vi "raster_scan_ground_shutter_new1.vi"() -> ()   [LabVIEW 2014] (continued)
{"X"=1085.0, "Y"=1.0008017239957097}, {"X"=1086.0, "Y"=1.0006641645030927}, {"X"=1087.0, "Y"=1.0004027285217332}, {"X"=1088.0, "Y"=1.0005489411934159}, {"X"=1089.0, "Y"=1.0007225000918056}, {"X"=1090.0, "Y"=1.0009034474609535}, {"X"=1091.0, "Y"=1.000700412495902}, {"X"=1092.0, "Y"=1.000559530919639}, {"X"=1093.0, "Y"=1.000504483593376}, {"X"=1094.0, "Y"=1.0006442407338632}, {"X"=1095.0, "Y"=1.0007664841012642}, {"X"=1096.0, "Y"=1.000595386528809}, {"X"=1097.0, "Y"=1.0006037218552855}, {"X"=1098.0, "Y"=1.0006076992023385}, {"X"=1099.0, "Y"=1.0008559458938961}, {"X"=1100.0, "Y"=1.0003974508855653}, {"X"=1101.0, "Y"=1.000520661832493}, {"X"=1102.0, "Y"=1.0007578111149742}, {"X"=1103.0, "Y"=1.0008950719357999}, {"X"=1104.0, "Y"=1.0005845587993554}, {"X"=1105.0, "Y"=1.0004975573787183}, {"X"=1106.0, "Y"=1.0005630280187985}, {"X"=1107.0, "Y"=1.0004865609128089}, {"X"=1108.0, "Y"=1.0005512637747156}, {"X"=1109.0, "Y"=1.0002904477140733}, {"X"=1110.0, "Y"=1.0007674753310123}, {"X"=1111.0, "Y"=1.00048425912666}, {"X"=1112.0, "Y"=1.000537310412031}, {"X"=1113.0, "Y"=1.0003184257671687}, {"X"=1114.0, "Y"=1.000551378960108}, {"X"=1115.0, "Y"=1.0004538385686341}, {"X"=1116.0, "Y"=1.0004718054037691}, {"X"=1117.0, "Y"=1.0005247856359447}, {"X"=1118.0, "Y"=1.000659286030276}, {"X"=1119.0, "Y"=1.0005952741982334}, {"X"=1120.0, "Y"=1.0003527948470332}, {"X"=1121.0, "Y"=1.0003785102284437}, {"X"=1122.0, "Y"=1.0003192400893162}, {"X"=1123.0, "Y"=1.0003699743364536}, {"X"=1124.0, "Y"=1.0004382463116217}, {"X"=1125.0, "Y"=1.0006464169345477}, {"X"=1126.0, "Y"=1.000249392202887}, {"X"=1127.0, "Y"=1.0003913257192574}, {"X"=1128.0, "Y"=1.0002131029939758}, {"X"=1129.0, "Y"=1.000510325890708}, {"X"=1130.0, "Y"=1.0003934905817833}, {"X"=1131.0, "Y"=1.0004037059793067}, {"X"=1132.0, "Y"=1.0006618492578454}, {"X"=1133.0, "Y"=1.0003001585452074}, {"X"=1134.0, "Y"=1.000318694948343}, {"X"=1135.0, "Y"=1.000487815893616}, {"X"=1136.0, "Y"=1.0003780216915208}, {"X"=1137.0, "Y"=1.000413317598835}, {"X"=1138.0, "Y"=1.0002135307505462}, {"X"=1139.0, "Y"=1.0003336207033005}, {"X"=1140.0, "Y"=1.000519988073343}, {"X"=1141.0, "Y"=1.000548679843787}, {"X"=1142.0, "Y"=1.000496056734601}, {"X"=1143.0, "Y"=1.0004444345976555}, {"X"=1144.0, "Y"=1.0001817232823744}, {"X"=1145.0, "Y"=1.000174005105797}, {"X"=1146.0, "Y"=1.000292447162328}, {"X"=1147.0, "Y"=1.0003638645546393}, {"X"=1148.0, "Y"=1.0002355752060164}, {"X"=1149.0, "Y"=1.00033455515827}, {"X"=1150.0, "Y"=1.0003245306564827}, {"X"=1151.0, "Y"=1.0002618152857234}, {"X"=1152.0, "Y"=1.0002737777366781}, {"X"=1153.0, "Y"=1.0002170643978059}, {"X"=1154.0, "Y"=1.000413604154719}, {"X"=1155.0, "Y"=1.0003099390465664}, {"X"=1156.0, "Y"=1.0005132182782912}, {"X"=1157.0, "Y"=1.000114107216987}, {"X"=1158.0, "Y"=1.0004770062354829}, {"X"=1159.0, "Y"=1.0004171034572575}, {"X"=1160.0, "Y"=1.0004569184938314}, {"X"=1161.0, "Y"=1.0004500384099237}, {"X"=1162.0, "Y"=1.0003170786145168}, {"X"=1163.0, "Y"=1.0002788252400026}, {"X"=1164.0, "Y"=1.0001948307072348}, {"X"=1165.0, "Y"=1.000410823030397}, {"X"=1166.0, "Y"=1.0004580665102198}, {"X"=1167.0, "Y"=1.0006692310587075}, {"X"=1168.0, "Y"=1.0003228737956749}, {"X"=1169.0, "Y"=1.0004916680510918}, {"X"=1170.0, "Y"=1.0003407364670853}, {"X"=1171.0, "Y"=1.0004045567333217}, {"X"=1172.0, "Y"=1.0003803654908978}, {"X"=1173.0, "Y"=1.0005615371076164}, {"X"=1174.0, "Y"=1.0004756109300434}, {"X"=1175.0, "Y"=1.0002314936984527}, {"X"=1176.0, "Y"=1.0004712973824592}, {"X"=1177.0, "Y"=1.0004057411969836}, {"X"=1178.0, "Y"=1.000628559692479}, {"X"=1179.0, "Y"=1.0003217635313526}, {"X"=1180.0, "Y"=1.0005789076417058}, {"X"=1181.0, "Y"=1.0004029462741326}, {"X"=1182.0, "Y"=1.0004755736162572}, {"X"=1183.0, "Y"=1.000328213200497}, {"X"=1184.0, "Y"=1.0003231498600846}, {"X"=1185.0, "Y"=1.000319103874417}, {"X"=1186.0, "Y"=1.0003228774765789}, {"X"=1187.0, "Y"=1.0003140546407656}, {"X"=1188.0, "Y"=1.0002848343336417}, {"X"=1189.0, "Y"=1.000508203882091}, {"X"=1190.0, "Y"=1.0002593068654488}, {"X"=1191.0, "Y"=1.000528935806764}, {"X"=1192.0, "Y"=1.0002378049460148}, {"X"=1193.0, "Y"=1.0005706812105148}, {"X"=1194.0, "Y"=1.0005374034632506}, {"X"=1195.0, "Y"=1.0001988163757602}, {"X"=1196.0, "Y"=1.0006119463054979}, {"X"=1197.0, "Y"=1.0004849225241381}, {"X"=1198.0, "Y"=1.0001640223128738}, {"X"=1199.0, "Y"=1.000498524564885}, {"X"=1200.0, "Y"=1.0004647778536588}, {"X"=1201.0, "Y"=1.000694727887658}, {"X"=1202.0, "Y"=1.0005207959941573}, {"X"=1203.0, "Y"=1.0004819931045297}, {"X"=1204.0, "Y"=1.000408028714742}, {"X"=1205.0, "Y"=1.000452772334067}, {"X"=1206.0, "Y"=1.0004315291178194}, {"X"=1207.0, "Y"=1.000614562289016}, {"X"=1208.0, "Y"=1.0004267608269495}, {"X"=1209.0, "Y"=1.0005413247966406}, {"X"=1210.0, "Y"=1.0003336212758853}, {"X"=1211.0, "Y"=1.0005233093467742}, {"X"=1212.0, "Y"=1.0001841951286268}, {"X"=1213.0, "Y"=1.000496276064622}, {"X"=1214.0, "Y"=1.0004435113554953}, {"X"=1215.0, "Y"=1.000312762889553}, {"X"=1216.0, "Y"=1.0003880506852765}, {"X"=1217.0, "Y"=1.0004430152993407}, {"X"=1218.0, "Y"=1.0005048604950806}, {"X"=1219.0, "Y"=1.0005918812246315}, {"X"=1220.0, "Y"=1.0005451398371954}, {"X"=1221.0, "Y"=1.0003538628812572}, {"X"=1222.0, "Y"=1.0002957581328165}, {"X"=1223.0, "Y"=1.0003455069942162}, {"X"=1224.0, "Y"=1.000559760984321}, {"X"=1225.0, "Y"=1.0006259813372131}, {"X"=1226.0, "Y"=1.0005780148556396}, {"X"=1227.0, "Y"=1.000428860631512}, {"X"=1228.0, "Y"=1.0003284274537925}, {"X"=1229.0, "Y"=1.0003759087401576}, {"X"=1230.0, "Y"=1.0004160325486642}, {"X"=1231.0, "Y"=1.000516966469858}, {"X"=1232.0, "Y"=1.0003531105538244}, {"X"=1233.0, "Y"=1.0003040660663642}, {"X"=1234.0, "Y"=1.0002145369130029}, {"X"=1235.0, "Y"=1.0006000845056313}, {"X"=1236.0, "Y"=1.0001780143915535}, {"X"=1237.0, "Y"=1.000413099776387}, {"X"=1238.0, "Y"=1.000340814364807}, {"X"=1239.0, "Y"=1.0003847961728747}, {"X"=1240.0, "Y"=1.0003377689644548}, {"X"=1241.0, "Y"=1.000235110479406}, {"X"=1242.0, "Y"=1.0003788090882357}, {"X"=1243.0, "Y"=1.0002683715599725}, {"X"=1244.0, "Y"=1.0005668734989672}, {"X"=1245.0, "Y"=1.0003983214098358}, {"X"=1246.0, "Y"=1.0004392908564488}, {"X"=1247.0, "Y"=1.0003490703578124}, {"X"=1248.0, "Y"=1.000515061423131}, {"X"=1249.0, "Y"=1.000536082836616}, {"X"=1250.0, "Y"=1.0006033938395056}, {"X"=1251.0, "Y"=1.000302436999363}, {"X"=1252.0, "Y"=1.0003435968686736}, {"X"=1253.0, "Y"=1.0003651518565015}, {"X"=1254.0, "Y"=1.0003753816897634}, {"X"=1255.0, "Y"=1.0004164707875218}, {"X"=1256.0, "Y"=1.0003124339083862}, {"X"=1257.0, "Y"=1.0006060617434724}, {"X"=1258.0, "Y"=1.0002433038607497}, {"X"=1259.0, "Y"=1.0005616162726159}, {"X"=1260.0, "Y"=1.0001358996051335}, {"X"=1261.0, "Y"=1.0004996326881244}, {"X"=1262.0, "Y"=1.000400823722666}, {"X"=1263.0, "Y"=1.0004651302016123}, {"X"=1264.0, "Y"=1.0004929661841928}, {"X"=1265.0, "Y"=1.000289786751315}, {"X"=1266.0, "Y"=1.0007068294577364}, {"X"=1267.0, "Y"=1.000512591719354}, {"X"=1268.0, "Y"=1.0005384306699427}, {"X"=1269.0, "Y"=1.000517410690437}, {"X"=1270.0, "Y"=1.0004457834676075}, {"X"=1271.0, "Y"=1.0003882566144624}, {"X"=1272.0, "Y"=1.000350183325496}, {"X"=1273.0, "Y"=1.0006835941128598}, {"X"=1274.0, "Y"=1.000354784112539}, {"X"=1275.0, "Y"=1.0005457804752032}, {"X"=1276.0, "Y"=1.0004234559458807}, {"X"=1277.0, "Y"=1.000496135909765}, {"X"=1278.0, "Y"=1.0002670384407588}, {"X"=1279.0, "Y"=1.0006040819275774}, {"X"=1280.0, "Y"=1.0002955765486259}, {"X"=1281.0, "Y"=1.000449882926412}, {"X"=1282.0, "Y"=1.000341046704705}, {"X"=1283.0, "Y"=1.0002621866108508}, {"X"=1284.0, "Y"=1.0002533451242017}, {"X"=1285.0, "Y"=1.0005020999666248}, {"X"=1286.0, "Y"=1.0004683221869657}, {"X"=1287.0, "Y"=1.0001189169044085}, {"X"=1288.0, "Y"=1.000394207742366}, {"X"=1289.0, "Y"=1.0004025113742172}, {"X"=1290.0, "Y"=1.0003591461387191}, {"X"=1291.0, "Y"=1.0002694424348582}, {"X"=1292.0, "Y"=1.000211944479205}, {"X"=1293.0, "Y"=1.0004554645660035}, {"X"=1294.0, "Y"=1.0004598057481355}, {"X"=1295.0, "Y"=1.0003228478676573}, {"X"=1296.0, "Y"=1.000281777127627}, {"X"=1297.0, "Y"=1.0003787502855446}, {"X"=1298.0, "Y"=1.0002643271177996}, {"X"=1299.0, "Y"=1.0003769449091497}, {"X"=1300.0, "Y"=1.0002871629718717}, {"X"=1301.0, "Y"=1.0002870790211043}, {"X"=1302.0, "Y"=1.0004704503723805}, {"X"=1303.0, "Y"=1.000476260657746}, {"X"=1304.0, "Y"=1.0004436163087576}, {"X"=1305.0, "Y"=1.0003863290955655}, {"X"=1306.0, "Y"=1.0005161647862937}, {"X"=1307.0, "Y"=1.0002249935131708}, {"X"=1308.0, "Y"=1.0005432839193034}, {"X"=1309.0, "Y"=1.0002816770022227}, {"X"=1310.0, "Y"=1.0004166737347884}, {"X"=1311.0, "Y"=1.000377784099795}, {"X"=1312.0, "Y"=1.000352088235326}, {"X"=1313.0, "Y"=1.0002378301300934}, {"X"=1314.0, "Y"=1.0004637548937716}, {"X"=1315.0, "Y"=1.0005468342453412}, {"X"=1316.0, "Y"=1.0002633492264565}, {"X"=1317.0, "Y"=1.000564439873648}, {"X"=1318.0, "Y"=1.0001624654733714}, {"X"=1319.0, "Y"=1.000511231090866}, {"X"=1320.0, "Y"=1.0003544601208683}, {"X"=1321.0, "Y"=1.0004053585602486}, {"X"=1322.0, "Y"=1.0004871315290047}, {"X"=1323.0, "Y"=1.0004300315929238}, {"X"=1324.0, "Y"=1.0003519445352231}, {"X"=1325.0, "Y"=1.0001932579752508}, {"X"=1326.0, "Y"=1.0004275604256458}, {"X"=1327.0, "Y"=1.0004909106276227}, {"X"=1328.0, "Y"=1.0003410593503033}, {"X"=1329.0, "Y"=1.0004439501902358}, {"X"=1330.0, "Y"=1.0005001161868323}, {"X"=1331.0, "Y"=1.0003332716770454}, {"X"=1332.0, "Y"=1.0005933376920328}, {"X"=1333.0, "Y"=1.0002798326870992}, {"X"=1334.0, "Y"=1.0004522633871564}, {"X"=1335.0, "Y"=1.0003822332936998}, {"X"=1336.0, "Y"=1.000511062012222}, {"X"=1337.0, "Y"=1.000358823903489}, {"X"=1338.0, "Y"=1.0006280323541772}, {"X"=1339.0, "Y"=1.00037812862855}]
  in  "# Images":u16=200 min=2 max=10000 step=2
  out "error out":errorcluster
  out "Camera Handle":u32=16842752
  out "Temperature":dbl=-75.5
  in  "error in":errorcluster
  # "Delay Stage Control"
  # "Calibration parameters"
  # "File Destination"
  # "Raster Scan Parameters"
  # "Microscope Stage Control"
  # "Fitting Parameters"
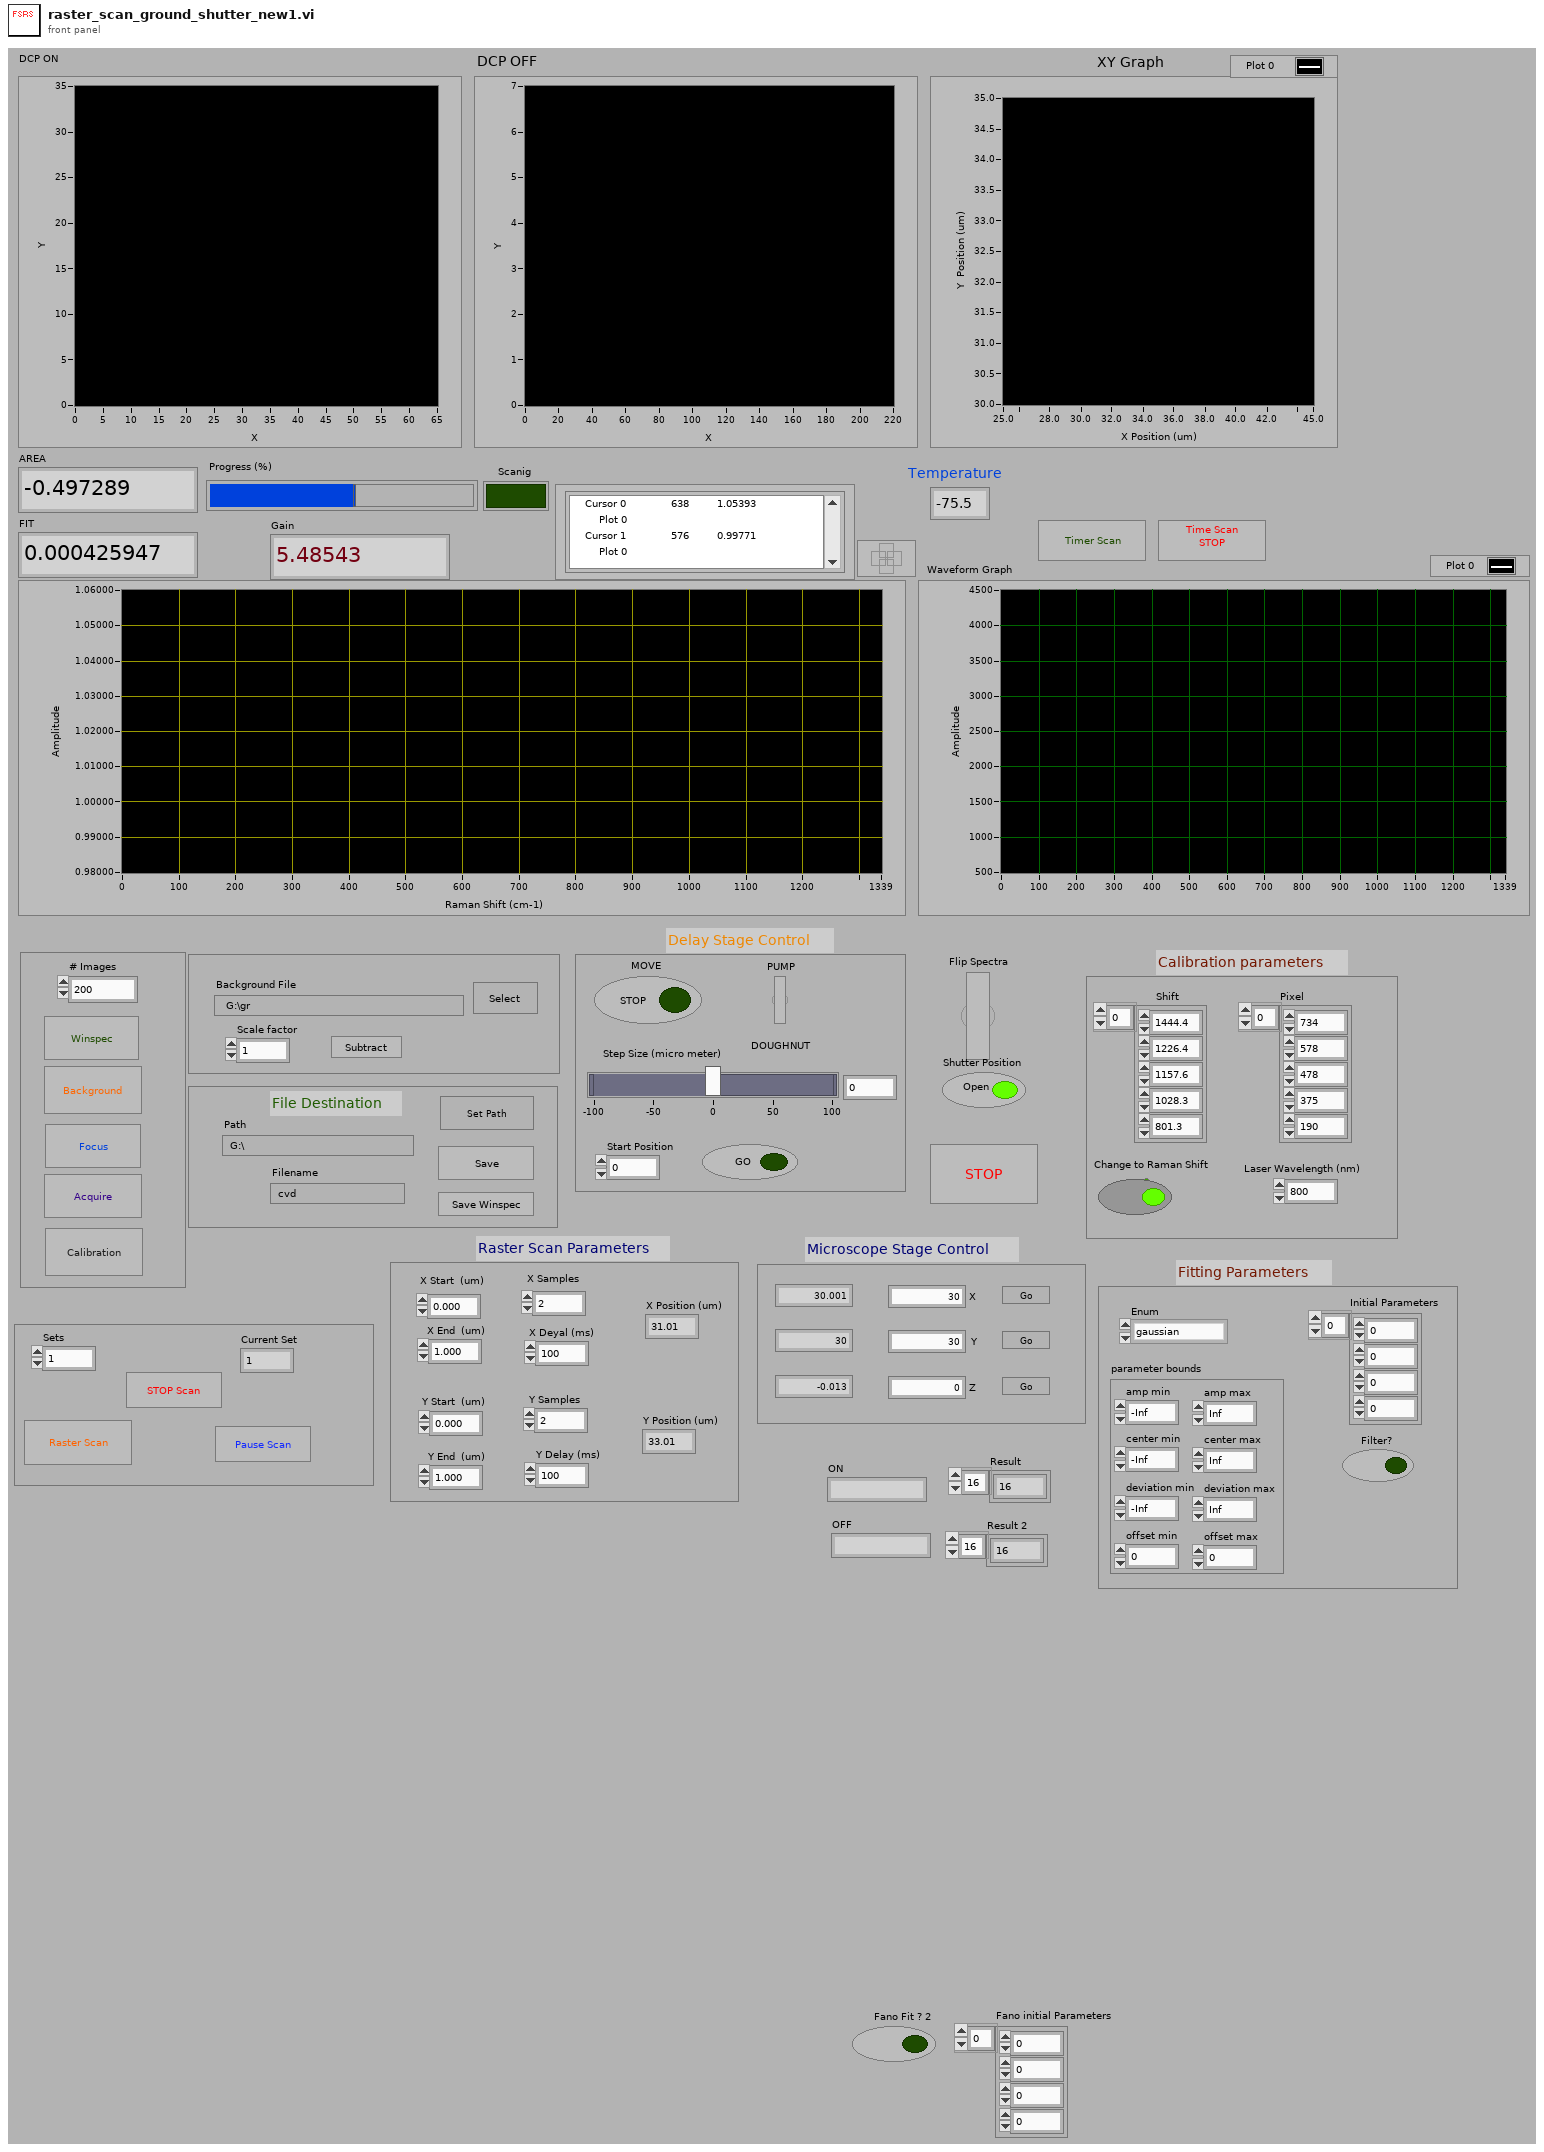
[diagram p1: front panel]
types:
  T1 = cluster{"amp min":dbl, "amp max":dbl, "center min":dbl, "center max":dbl, "deviation min":dbl, "deviation max":dbl, "offset min":dbl, "offset max":dbl}
  T2 = typedef "Control 2.ctl" = dbl[]
  T3 = enum8{"Enabled", "Disabled", "Disabled and Grayed Out"}
  T4 = cluster{"X start":u32, "X end":u32, "X Binning/Grouping":u32, "Y start":u32, "Y end":u32, "Y Binning/Grouping":u32}
  T5 = cluster{dbl[][], dbl[][], dbl[][], dbl[][], bool}
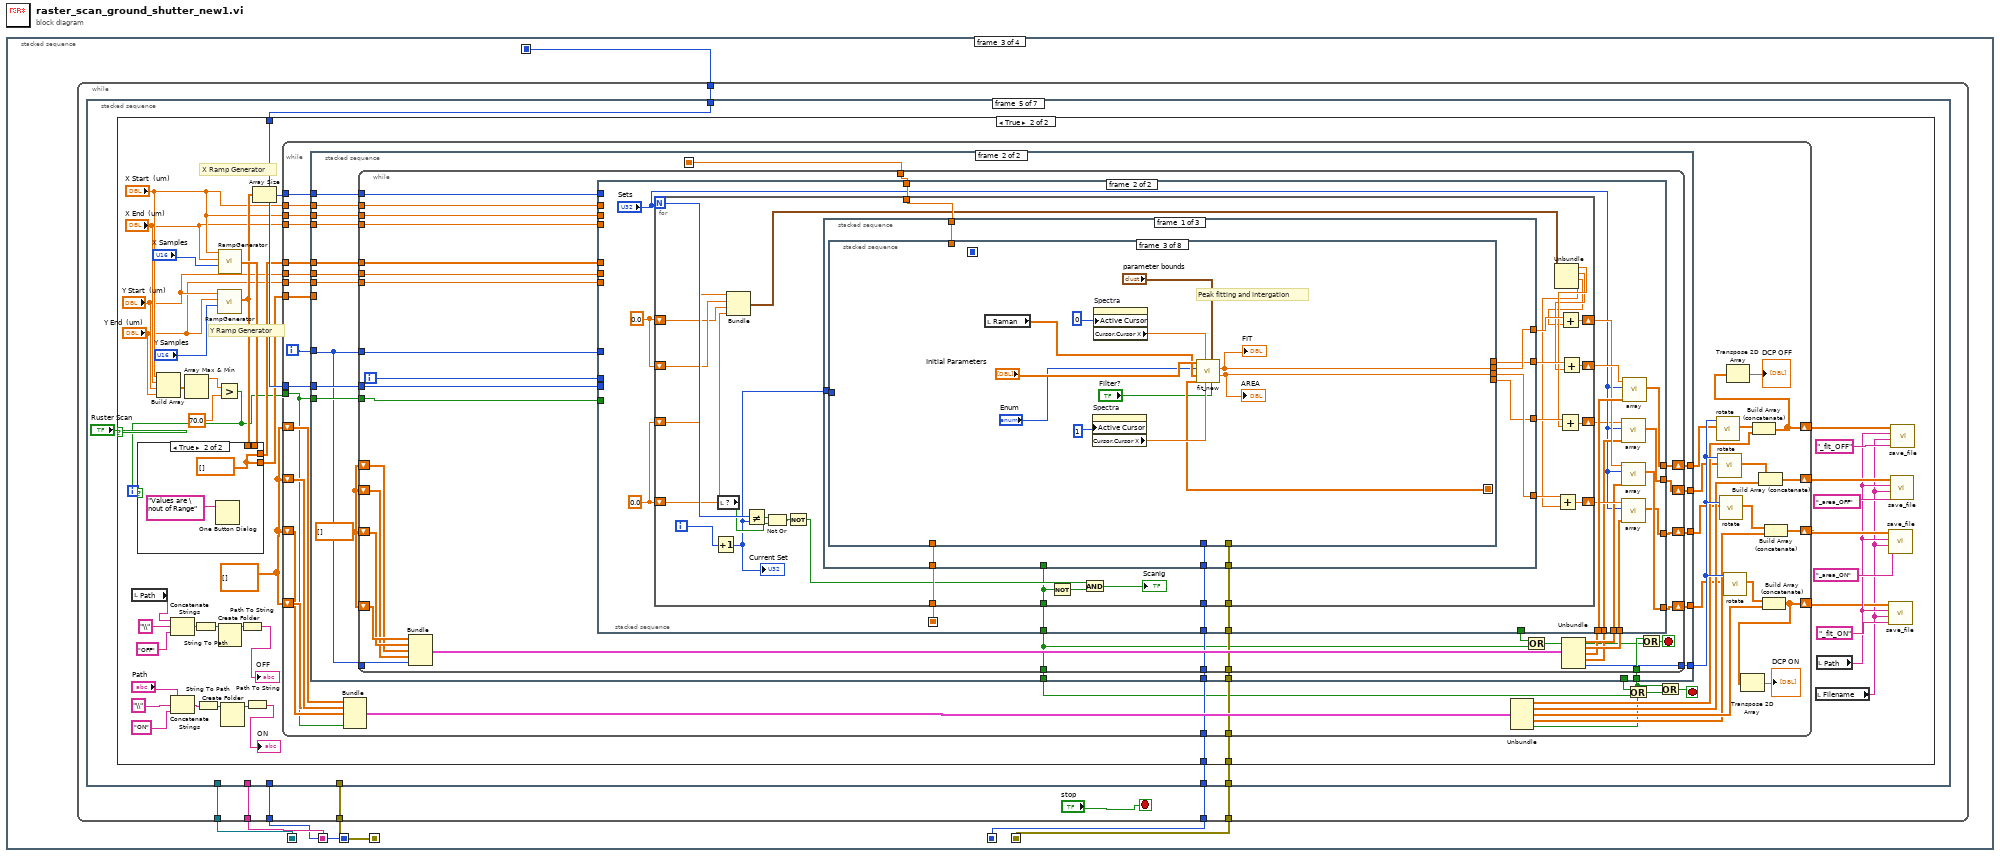
[diagram p0: block diagram]
diagram:
  n1 = stacked-sequence {
    seq-local: [w18 _ _ _] -> [_ _ w119 _]
    seq-local: [w17 _ _ _] -> [_ _ w118 _]
    seq-local: [w16 _ _ _] -> [_ _ w117 _]
    seq-local: [w15 _ _ _] -> [_ _ w116 _]
    seq-local: [w14 _ _ _] -> [_ _ w115 w864]
    seq-local: [w13 _ _ _] -> [_ _ w114 _]
    seq-local: [w12 _ _ _] -> [_ _ w113 _]
    frame #0 {
      w10 = 1340
      w76 = 0
      w78 = 8
      # "4: shutter opened while waiting for trigger\n3: Shutter opened during entire acq sequence\n2:Shutter opened and closed for each exposure\n\nOther numbers: Time in ms to open and close"
      # "1 is for free run, 3 ext sync"
      # "Parameter id settings:\n119: enable custon timing for horizontal and vertical shift\n121:Parallel shift time override\n146: Skip serial register clean\n 4:  Set logic output to \"Not Ready\" (necessary for chopper sync)"
      # "Setting up the PIXIS and all the environment variables\nHave Renee fill in the rest."
      n2 = call "ExSubInitNOpenCam.vi"("error in (no error)"="error in") -> ("Camera Handle"=w91:u32, "error out"=w48:errorcluster)
      n3 = call <userlib>:"CameraGetDataDim.vi"("Camera Handle"=w91, "error in"=w48) -> ("Camera Handle"=w88:u32, "Xdim"=w90:u32, "Ydim"=w89:u32, "error out"=w87:errorcluster)
      n4 = global write "MaxX.vi" "X Max in"(w90) -> ()
      n5 = global write "MaxY.vi" "Max Y in"(w89) -> ()
      n6 = call "pico_init.vi"() -> ("error out 3"=w15:errorcluster, "ID"=w16:i32, "key"=w17:string, "CmdLib Out"=w18:refnum<k24>)  [unwired: 8 in]
      n7 = call <userlib>:"CameraSetTemp.vi"("error in (no error)"=w87, "Temperature"=-75, "Camera Handle"=w88) -> ("error out"=w84:errorcluster, "Camera Handle"=w85:u32)
      n8 = call <userlib>:"CameraADCset.vi"("ADC offset"=0, "Read Out port"=2, "error in (no error)"=w84, "ADC Gain"=1, "ADC Speed"=-2, "Camera Handle"=w85) -> ("error out"=w79:errorcluster, "Camera Handle"=w80:u32)
      n9 = Bundle(w78, w78, 100, w76, w76, w10) -> (w75:cluster{i32, i32, i32, i32, i32, i32})  [unwired: 1 in]
      n10 = call <userlib>:"CameraSetCustomChip.vi"("error in (no error)"=w79, "Custom Chip Settings"=w75, "Enable/Disable Custom Chip"=TRUE, "Camera Handle"=w80) -> ("error out"=w72:errorcluster, "Camera Handle"=w73:u32)
      n11 = call <userlib>:"CameraSkips.vi"("Camera Handle"=w73, "Minimum Block Size"=100, "Number of Minimum blocks"=1, "error in"=w72, "Type of Skips"=1) -> ("Camera Handle"=w67:u32, "error out"=w68:errorcluster)
      n12 = call "StandardInit.vi"() -> ("Outgoing Handle"=w14:i32)  [unwired: 1 in]
      n13 = call <userlib>:"CameraCleans.vi"("Camera Handle"=w67, "Number of Clears"=1, "Number of Strips Per Clear"=100, "error in"=w68, "Continuous Clears"=0) -> ("Camera Handle"=w62:u32, "error out"=w63:errorcluster)
      n14 = call <userlib>:"CameraTrigger.vi"("error in"=w63, "Trigger Edge"=1, "Timing Mode"=3, "Camera Handle"=w62) -> ("error out"=w40:errorcluster, "Camera Handle"=w39:u32)
      n15 = Bundle By Name(cluster=T4 {"X start"=0, "X end"=0, "X Binning/Grouping"=0, "Y start"=0, "Y end"=0, "Y Binning/Grouping"=0} ("ROI Params"), "X start"=u32 1, "X end"=u32 1340, "X Binning/Grouping"=u32 1, "Y start"=u32 1, "Y end"=u32 100, "Y Binning/Grouping"=u32 100) -> (w21:T4)
      n16 = call <userlib>:"CameraROI.vi"("error in"=w40, "ROI Params"=w21, "ROI Index"=1, "Camera Handle"=w39) -> ("error out"=w34:errorcluster, "Camera Handle"=w33:u32)
      n17 = call <userlib>:"CameraShutter.vi"("Camera Handle"=w33, "Shutter Comp Time: Pre Open"=0, "Shutter Comp Time: Post Open"=0, "error in"=w34, "Shutter State"=3) -> ("Camera Handle"=w32:u32, "error out"=w23:errorcluster)
      n18 = call <userlib>:"CameraSetVar.vi"("error in"=w23, "Value"=1.0, "Parameter ID"=119, "Camera Handle"=w32) -> ("error out"=w57:errorcluster, "CameraHandle"=w55:u32)
      n19 = call <userlib>:"CameraSetVar.vi"("error in"=w57, "Value"=3200.0, "Parameter ID"=121, "Camera Handle"=w55) -> ("error out"=w56:errorcluster, "CameraHandle"=w54:u32)
      n20 = call <userlib>:"CameraSetVar.vi"("error in"=w56, "Value"=1.0, "Parameter ID"=146, "Camera Handle"=w54) -> ("error out"=w28:errorcluster, "CameraHandle"=w27:u32)
      n21 = call <userlib>:"CameraSetVar.vi"("error in"=w28, "Value"=3.0, "Parameter ID"=4, "Camera Handle"=w27) -> ("error out"=w26:errorcluster, "CameraHandle"=w19:u32)
      n22 = call <userlib>:"ToolKitIsError.vi"("error in"=w26, "Reserved"=w19) -> ("error out"=w58:errorcluster, "Error Flag"=w59:bool)
      n23 = case shown="False" w59 {
        tunnel: w58 -> [_ w103]
        tunnel: [w102 w103] -> w20
        tunnel: w48 -> [w102 _]
        frame False {
        }
        frame True {
        }
      }
      n24 = while {
        tunnel: w20 -> [w100]
        tunnel: [w99] -> w36
        tunnel: w19 -> [w98]
        tunnel: [w97] -> w37
        stop <- w95 continue-if-true
        # "This loop makes sure the camera has cooled down completely"
        n25 = call <userlib>:"CameraGetTemp.vi"("Camera Handle"=w98, "error in (no error)"=w100) -> ("Camera Handle"=w97:u32, "Temperature"=w94:dbl, "error out"=w99:errorcluster)
        "Temperature" <- w94
        n26 = Wait Until Next ms Multiple(millisecond multiple=1000 ("ADC Gain")) -> ()  [unwired: 1 out]
        n27 = Greater?(x=w94, y=-75) -> (0:w95:bool)
      }
      "Camera Handle" <- w37
      "error out" <- w36
      n28 = for {
        N: w10 -> [_]
        tunnel: [w93] -> w11 mode=indexing
        i -> [w93]
      }
      n29 = local write "Result 2"(w11) -> ()
      n30 = local write "Result"(w11) -> ()
      n31 = call "Shutter_Init.vi"() -> ("error out"=w12:errorcluster, "ObjectPtr"=w13:i32)  [unwired: 2 in]
      n32 = property on="Callibration" class="Bool"("DisabledEnum"=T3."Disabled and Grayed Out" ("Disabled")) -> ()  [unwired: 2 in, 2 out]
      n33 = property on="Pause" class="Bool (strict)"("DisabledEnum"=T3."Disabled and Grayed Out" ("Disabled")) -> ()  [unwired: 2 in, 2 out]
      n34 = property on="winspec" class="Bool (strict)"("DisabledEnum"=T3."Disabled and Grayed Out" ("Disabled")) -> ()  [unwired: 2 in, 2 out]
      n35 = property on="Ruster Scan" class="Bool"("DisabledEnum"=T3."Disabled and Grayed Out" ("Disabled")) -> ()  [unwired: 2 in, 2 out]
      n36 = property on="Acquire" class="Bool"("DisabledEnum"=T3."Disabled and Grayed Out" ("Disabled")) -> ()  [unwired: 2 in, 2 out]
      n37 = property on="stop" class="Bool"("DisabledEnum"=T3."Disabled and Grayed Out" ("Disabled")) -> ()  [unwired: 2 in, 2 out]
      n38 = property on="STOP Scan" class="Bool"("DisabledEnum"=T3."Disabled and Grayed Out" ("Disabled")) -> ()  [unwired: 2 in, 2 out]
      n39 = property on="Focus" class="Bool (strict)"("DisabledEnum"=T3."Disabled and Grayed Out" ("Disabled")) -> ()  [unwired: 2 in, 2 out]
      n40 = property on="Bkgnd" class="Bool"("DisabledEnum"=T3."Disabled and Grayed Out" ("Disabled")) -> ()  [unwired: 2 in, 2 out]
    }
    frame #1 {
      n41 = property on="STOP Scan" class="Bool"("DisabledEnum"=T3."Enabled" ("Disabled")) -> ()  [unwired: 2 in, 2 out]
      n42 = property on="Pause" class="Bool (strict)"("DisabledEnum"=T3."Enabled" ("Disabled")) -> ()  [unwired: 2 in, 2 out]
      n43 = property on="stop" class="Bool"("DisabledEnum"=T3."Enabled" ("Disabled")) -> ()  [unwired: 2 in, 2 out]
      n44 = property on="Bkgnd" class="Bool"("DisabledEnum"=T3."Enabled" ("Disabled")) -> ()  [unwired: 2 in, 2 out]
      n45 = property on="Ruster Scan" class="Bool"("DisabledEnum"=T3."Enabled" ("Disabled")) -> ()  [unwired: 2 in, 2 out]
      n46 = property on="winspec" class="Bool (strict)"("DisabledEnum"=T3."Enabled" ("Disabled")) -> ()  [unwired: 2 in, 2 out]
      n47 = property on="Focus" class="Bool (strict)"("DisabledEnum"=T3."Enabled" ("Disabled")) -> ()  [unwired: 2 in, 2 out]
      n48 = property on="Acquire" class="Bool"("DisabledEnum"=T3."Enabled" ("Disabled")) -> ()  [unwired: 2 in, 2 out]
      n49 = property on="Callibration" class="Bool"("DisabledEnum"=T3."Enabled" ("Disabled")) -> ()  [unwired: 2 in, 2 out]
    }
    frame #2 {
      n50 = while {
        tunnel: w119 -> [w127]
        tunnel: w118 -> [w126]
        tunnel: w117 -> [w125]
        tunnel: w116 -> [w124]
        tunnel: w115 -> [w123]
        tunnel: w114 -> [w122]
        tunnel: w113 -> [w121]
        stop <- "stop" stop-if-true
        n51 = stacked-sequence {
          tunnel: w127 -> [w133 _ _ w229 _ _ _]
          tunnel: w126 -> [w132 _ _ w228 _ _ _]
          tunnel: w125 -> [w130 _ _ w227 _ _ _]
          tunnel: w124 -> [w131 _ _ w226 _ _ _]
          tunnel: w123 -> [_ _ _ w223 w358 _ _]
          tunnel: w122 -> [w129 _ _ w222 w357 _ _]
          tunnel: w121 -> [w128 _ _ w221 w356 _ _]
          frame #0 {
            n52 = case shown="True" "winspec" {
              tunnel: w133 -> [_ w142]
              tunnel: w132 -> [_ w141]
              tunnel: w131 -> [_ w139]
              tunnel: w130 -> [_ w138]
              tunnel: w129 -> [_ w136]
              tunnel: w128 -> [_ w135]
              frame False {
              }
              frame True {
                n53 = while {
                  tunnel: w142 -> [w147]
                  tunnel: w141 -> [w148]
                  tunnel: w139 -> [w156]
                  tunnel: w138 -> [w149]
                  stop <- w163 continue-if-true
                  n54 = stacked-sequence {
                    frame #0 {
                      # "This loop continuously updates the graph on the front with the image from the PIXIS"
                      n55 = local read "Camera Handle"() -> (w178:u32)
                      n56 = local read "# Images"() -> (w174:u16)
                      n57 = local read "error out"() -> (w177:errorcluster)
                      n58 = local read "Change to Raman Shift"() -> (w168:bool)
                      n59 = call "DataGrabber.vi"("# Images In"=w174, "Camera Handle"=w178, "error in (no error)"=w177) -> ("# Images Out"=w169:u16, "Camera Handle"=w176:u32, "Data"=w173:dbl[][], "error out"=w175:errorcluster)
                      n60 = case shown="True" w168 {
                        tunnel: [w180 w182] -> w166
                        tunnel: ["Pixel" ("X Scale.Name Label.Text") "Raman Shift (cm-1)" ("X Scale.Name Label.Text")] -> w164
                        frame False {
                          n61 = local read "Result"() -> (w180:dbl[])
                        }
                        frame True {
                          n62 = local read "Result 2"() -> (w182:dbl[])
                        }
                      }
                      n63 = Initialize Array(0.0, u32 1340) -> (w170:dbl[])
                      n64 = call "DataProcessor.vi"("PumpOffBkgd"=w170, "PumpOnBkgd"=w170, "Data"=w173, "# of Images"=w169) -> ("PumpOff"=w167:dbl[])  [unwired: 2 out]
                      n65 = local write "# Images"(w169) -> ()
                      n66 = Build Cluster Array(w166, w167) -> (w165:cluster{dbl, dbl}[])
                      n67 = property on="Spectra" class="XYGraph (strict)"("XScale.NameLbl.Text"=w164) -> ()  [unwired: 2 in, 2 out]
                      n68 = local write "Spectra"(w165) -> ()
                      n69 = local write "Camera Handle"(w176) -> ()
                      n70 = local write "error out"(w175) -> ()
                    }
                    frame #1 {
                      n71 = stacked-sequence {
                        frame #0 {
                          # "Select Cursor 0"
                          n72 = property on="Spectra" class="XYGraph (strict)"("Active Cursor"=0) -> ()  [unwired: 2 in, 2 out]
                        }
                        frame #1 {
                          # "Record the Y position of cursor 0"
                        }
                        frame #2 {
                          # "Select Cursor 1"
                          n73 = property on="Spectra" class="XYGraph (strict)"("Active Cursor"=1) -> ()  [unwired: 2 in, 2 out]
                        }
                        frame #3 {
                          # "Calculate the Gain"
                          n74 = property on="Spectra" class="XYGraph (strict)"() -> ("Cursor.Cursor Position:Cursor Y"=w190:dbl)  [unwired: 2 in, 2 out]
                          n75 = local read "cursor y 2"() -> (w189:dbl)
                          n76 = Subtract(x=w190, y=w189) -> (x-y=w186:dbl)
                          n77 = Absolute Value(x=w186) -> (abs(x)=w188:dbl)
                          n78 = Multiply(x=w188, y=1) -> (x*y=w185:dbl)
                          n79 = local write "Gain"(w185) -> ()
                        }
                      }
                    }
                  }
                  n80 = local read "winspec"() -> (w163:bool)
                  n81 = Boolean To (0,1)(Boolean="PUMP") -> (0, 1=w161:i16)
                  n82 = Multiply(x="Step Size (micro meter)", y=10.0) -> (x*y=w144:dbl)
                  n83 = Add(x=w161, y=i16 1) -> (x+y=w150:i16)
                  n84 = Round To Nearest(number=w144) -> (nearest integer value=w143:dbl)
                  n85 = And(x="MOVE", y=w163) -> (x .and. y?=w157:bool)
                  n86 = call "Pico_move_new.vi"("Motor"=w150, "CmdLib Out"=w147, "DeviceKey Out"=w148, "Start Position"="Start Position", "Boolean 2"="GO", "Relative Steps"=w143, "Boolean"=w157, "error out"=w156, "Device Address Out"=w149) -> ("CmdLib Out"=→"CmdLib Out":refnum<k24>, "DeviceKey Out"=→"DeviceKey Out":string, "Device Address Out"=→"Device Address Out":i32, "error out 2"=→"error out 2":errorcluster)  [unwired: 3 in]
                }
                n87 = call "shutter_new.vi"("error in"=w135, "ShutterID"=310, "Shutter Position"="Shutter Position", "ObjectPtr"=w136) -> ()  [unwired: 1 out]
              }
            }
          }
          frame #1 {
            n88 = case shown="True" "Bkgnd" {
              frame False {
              }
              frame True {
                # "Process the Data"
                # "Get the data!"
                # "Display the Raman Pump on graph on the Front Panel and store data"
                n89 = local read "Camera Handle"() -> (w205:u32)
                n90 = local read "# Images"() -> (w200:u16)
                n91 = local read "error out"() -> (w204:errorcluster)
                n92 = local read "Change to Raman Shift"() -> (w193:bool)
                n93 = call "DataGrabber.vi"("# Images In"=w200, "Camera Handle"=w205, "error in (no error)"=w204) -> ("# Images Out"=w197:u16, "Camera Handle"=w203:u32, "Data"=w201:dbl[][], "error out"=w202:errorcluster)
                n94 = local write "Camera Handle"(w203) -> ()
                n95 = local write "error out"(w202) -> ()
                n96 = local write "# Images"(w197) -> ()
                n97 = case shown="True" w193 {
                  tunnel: [w209 w211] -> w196
                  tunnel: ["Pixel" ("X Scale.Name Label.Text") "Raman Shift (cm-1)" ("X Scale.Name Label.Text")] -> w192
                  frame False {
                    n98 = local read "Result"() -> (w209:dbl[])
                  }
                  frame True {
                    n99 = local read "Result 2"() -> (w211:dbl[])
                  }
                }
                n100 = Initialize Array(0.0) -> (w198:dbl[])  [unwired: 1 in]
                n101 = call "DataProcessor.vi"("PumpOffBkgd"=w198, "PumpOnBkgd"=w198, "Data"=w201, "# of Images"=w197) -> ("PumpOff"=→"Bkgndoff":dbl[], "PumpOn"=→"Bkgndon":dbl[], "Raman"=w195:dbl[])
                n102 = Build Cluster Array(w196, w195) -> (w194:cluster{dbl, dbl}[])
                n103 = property on="Spectra" class="XYGraph (strict)"("XScale.NameLbl.Text"=w192) -> ()  [unwired: 2 in, 2 out]
                n104 = local write "Spectra"(w194) -> ()
              }
            }
          }
          frame #2 {
            n105 = case shown="True" "Callibration" {
              frame False {
              }
              frame True {
                n106 = for {
                  N: 1340 -> [_]
                  tunnel: [w220] -> w219 mode=indexing
                  i -> [w220]
                }
                n107 = call "cal.vi"("array"=w219, "Laser Wavelength"="Laser Wavelength (nm)", "Wave Number"="Shift", "Pixel"="Pixel") -> ("array 2"=→"Result":dbl[], "Result"=→"Result 2":dbl[])  [unwired: 6 in]
              }
            }
          }
          frame #3 {
            n108 = Compound Arithmetic op=OR("Acquire", "Focus") -> (w230:bool)
            n109 = case shown="True" w230 {
              selector: w230 -> [_ w238]
              tunnel: w229 -> [_ w237]
              tunnel: w228 -> [_ w236]
              tunnel: w227 -> [_ w235]
              tunnel: w226 -> [_ w234]
              tunnel: w223 -> [_ w233]
              tunnel: w222 -> [_ w232]
              tunnel: w221 -> [_ w231]
              frame False {
              }
              frame True {
                n110 = while {
                  tunnel: w238 -> [w276]
                  tunnel: w237 -> [w268]
                  tunnel: w236 -> [w267]
                  tunnel: w235 -> [w266]
                  tunnel: w234 -> [w265]
                  tunnel: w233 -> [w244]
                  tunnel: w232 -> [w240]
                  tunnel: w231 -> [w239]
                  stop <- w243 continue-if-true
                  n111 = stacked-sequence {
                    seq-local: [w288 _ _ _] -> [_ w311 _ _]
                    seq-local: [w293 _ _ _] -> [_ w308 _ _]
                    frame #0 {
                      n112 = local read "Camera Handle"() -> (w297:u32)
                      n113 = local read "# Images"() -> (w298:u16)
                      n114 = local read "error out"() -> (w296:errorcluster)
                      n115 = local read "Change to Raman Shift"() -> (w284:bool)
                      n116 = call "DataGrabber.vi"("# Images In"=w298, "Camera Handle"=w297, "error in (no error)"=w296) -> ("# Images Out"=w288:u16, "Camera Handle"=w294:u32, "Data"=w293:dbl[][], "error out"=w295:errorcluster)
                      n117 = case shown="False" w284 {
                        tunnel: [w300 w302] -> w282
                        tunnel: ["Pixel" ("X Scale.Name Label.Text") "Raman Shift (cm-1)" ("X Scale.Name Label.Text")] -> w285
                        frame False {
                          n118 = local read "Result"() -> (w300:dbl[])
                        }
                        frame True {
                          n119 = local read "Result 2"() -> (w302:dbl[])
                        }
                      }
                      n120 = local write "Camera Handle"(w294) -> ()
                      n121 = local write "error out"(w295) -> ()
                      n122 = Initialize Array(0.0, u32 1340) -> (w290:dbl[])
                      n123 = call "DataProcessor.vi"("PumpOffBkgd"=w290, "PumpOnBkgd"=w290, "Data"=w293, "# of Images"=w288) -> ("PumpOff"=w280:dbl[], "PumpOn"=w289:dbl[], "Raman"=w286:dbl[])
                      n124 = local write "# Images"(w288) -> ()
                      n125 = local write "Waveform Graph"(w280) -> ()
                      n126 = property on="Spectra" class="XYGraph (strict)"("XScale.NameLbl.Text"=w285) -> ()  [unwired: 2 in, 2 out]
                      n127 = local write "On"(w289) -> ()
                      n128 = local write "Off"(w280) -> ()
                      n129 = case shown="True" "Flip Spectra" {
                        tunnel: [w303 w304] -> w283
                        tunnel: w286 -> [w303 w305]
                        frame False {
                        }
                        frame True {
                          # "Flip Displayed Spectra"
                          n130 = Reciprocal(x=w305) -> (1/x=w304:dbl[])
                        }
                      }
                      n131 = local write "Raman"(w286) -> ()
                      n132 = Build Cluster Array(w282, w283) -> (w281:cluster{dbl, dbl}[])
                      n133 = local write "Spectra"(w281) -> ()
                    }
                    frame #1 {
                      w315 = 2
                      n134 = Initialize Array(0.0, u32 1340) -> (w319:dbl[])
                      n135 = Initialize Array(0.0, u32 1340) -> (w320:dbl[])
                      n136 = Subtract(x=w311, y=u16 10) -> (x-y=w310:u16)
                      n137 = Divide(x=w311, y=w315) -> (x/y=w316:dbl)
                      n138 = Delete From Array(array=w308, length=10, index (row)=0) -> (array with subset deleted=w307:dbl[][])  [unwired: 1 in, 1 out]
                      n139 = for {
                        N: w310 -> [_]
                        tunnel: w307 -> [w331]
                        shift-right: [w329] -> w318
                        shift-left: w320 -> [w330]
                        shift-right: [w327] -> w317
                        shift-left: w319 -> [w328]
